vi "kinectRead [ColorFrame].vi"(8 "error in (no error)":errorcluster, 9 "Timeout (ms)":i32=5000, 11 "KinectSensor References in":T1) -> (0 "error out":errorcluster, 2 "frameData":u8[](array[numeric]), 3 "KinectSensor References out":T1)   [LabVIEW 2014]
uses:
  controls/KinectSensor References.ctl
  Microsoft.Kinect
  C:/github/labviewhacker/LVH-KinectOne/LabVIEW/vi.lib/LabVIEW Hacker/KinectOne/support/BodyFrameDataInterface.dll
  BodyFrameDataInterface.dll
  Frame Data FGV [Color].vi
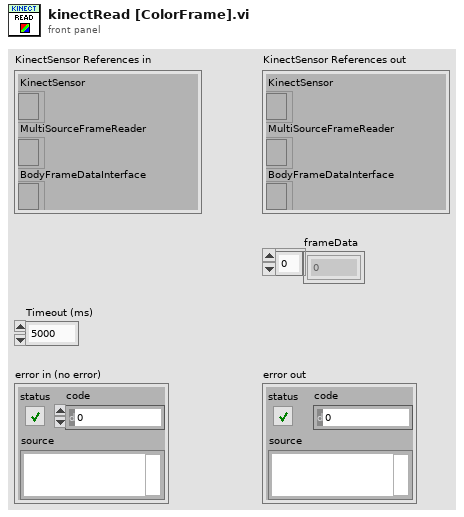
[diagram p1: front panel]
types:
  T1 = typedef "KinectSensor References.ctl" = cluster{"KinectSensor":refnum<k24>, "MultiSourceFrameReader":refnum<k24>, "BodyFrameDataInterface":refnum<k24>}
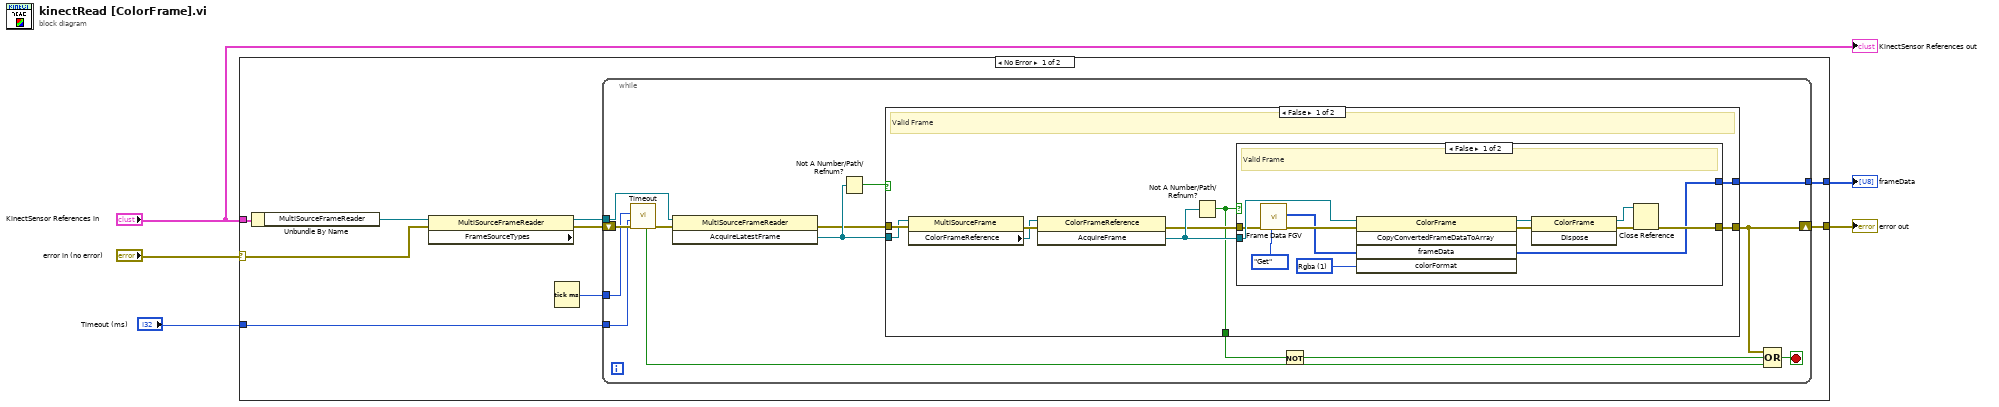
[diagram p0: block diagram]
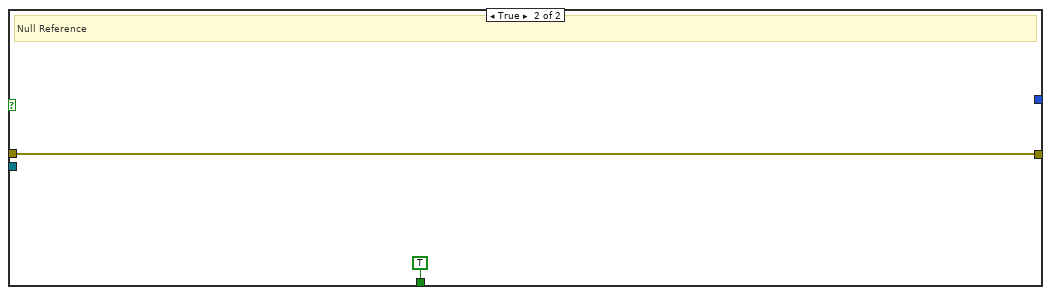
[diagram p3: hidden frame]
diagram:
  n1 = case shown="No Error" "error in (no error)" {
    selector: "error in (no error)" -> [w6 w53]
    tunnel: "KinectSensor References in" -> [w11 _]
    tunnel: [w10 w53] -> w4
    tunnel: [w9 _] -> w3
    tunnel: "Timeout (ms)" -> [w7 _]
    frame No Error {
      n2 = Unbundle By Name(w11) -> ("MultiSourceFrameReader"=w12:refnum<k24>)
      n3 = property class="MultiSourceFrameReader" props=["FrameSourceTypes"](reference=w12, error in=w6) -> (reference out=w14:refnum<k24>, error out=w13:errorcluster)  [unwired: 1 out]
      n4 = Tick Count (ms)() -> (millisecond timer value=w8:u32)
      n5 = while {
        tunnel: w14 -> [w22]
        shift-right: [w19] -> w10
        shift-left: w13 -> [w24]
        tunnel: [w25] -> w9
        tunnel: w8 -> [w21]
        tunnel: w7 -> [w20]
        stop <- w18 stop-if-true
        n6 = call "Timeout.vi"("error in (no error)"=w24, "Timeout (ms)"=w20, "Start Time"=w21) -> ("error out"=w23:errorcluster, "Timeout?"=w15:bool)  [unwired: 7 in]
        n7 = invoke class="MultiSourceFrameReader" method="AcquireLatestFrame"(reference=w22, error in=w23) -> (error out=w27:errorcluster, "AcquireLatestFrame"=w28:refnum<k24>)  [unwired: 1 in, 1 out]
        n8 = Not A Number/Path/Refnum?(number/path/refnum=w28) -> (NaN/Path/Refnum?=w26:bool)
        n9 = case shown="False" w26 {
          tunnel: w27 -> [w34 w51]
          tunnel: w28 -> [w31 _]
          tunnel: [w33 w51] -> w19
          tunnel: [w32 TRUE] -> w17
          tunnel: [w29 _] -> w25
          frame False {
            # "Valid Frame"
            n10 = property class="MultiSourceFrame"(reference=w31, error in=w34) -> (error out=w35:errorcluster, "ColorFrameReference"=w30:refnum<k24>)  [unwired: 1 out]
            n11 = invoke class="ColorFrameReference" method="AcquireFrame"(reference=w30, error in=w35) -> (error out=w36:errorcluster, "AcquireFrame"=w37:refnum<k24>)  [unwired: 1 in, 1 out]
            n12 = Not A Number/Path/Refnum?(number/path/refnum=w37) -> (NaN/Path/Refnum?=w32:bool)
            n13 = case shown="False" w32 {
              tunnel: w36 -> [w41 w50]
              tunnel: w37 -> [w44 _]
              tunnel: [w43 w50] -> w33
              tunnel: [w42 _] -> w29
              frame False {
                w45 = 1 items=["None", "Rgba", "Yuv", "Bgra", "Bayer", "Yuy2"] ("colorFormat")
                # "Valid Frame"
                n14 = call-poly "Frame Data FGV.vi"("Command"=enum16{"Get", "Initialize"}."Get", "error in (no error)"=w41) -> ("error out"=w40:errorcluster, "Byte Array"=w39:u8[])  [unwired: 8 in]
                n15 = invoke class="ColorFrame" method="CopyConvertedFrameDataToArray"(reference=w44, error in=w40, "frameData"=w39, "colorFormat"=w45) -> (reference out=w46:refnum<k24>, error out=w47:errorcluster, "frameData"=w42:u8[])  [unwired: 1 in, 2 out]
                n16 = invoke class="ColorFrame" method="Dispose"(reference=w46, error in=w47) -> (reference out=w49:refnum<k24>, error out=w48:errorcluster)  [unwired: 1 in, 1 out]
                n17 = Close Reference(reference=w49, error in (no error)=w48) -> (error out=w43:errorcluster)
              }
              frame True {
                # "Null Reference"
              }
            }
          }
          frame True {
            # "Null Reference"
          }
        }
        n18 = Not(x=w17) -> (.not. x?=w16:bool)
        n19 = Compound Arithmetic op=OR(w19, w16, w15) -> (w18:bool)
      }
    }
    frame Error {
    }
  }
  "error out" <- w4
  "frameData" <- w3
  "KinectSensor References out" <- "KinectSensor References in"
